vi "BG_move.vi"(4 "Reset_x":i32, 6 "Return_x":i32, 7 "Mov_Spd":i32, 8 "error in":errorcluster, 11 "BG_ref":refnum<vi>[](array[refnum])) -> (0 "error out":errorcluster)   [LabVIEW 8.6]
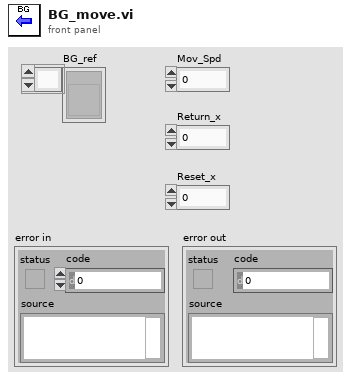
[diagram p1: front panel]
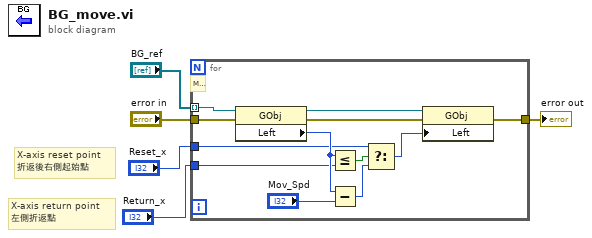
[diagram p0: block diagram]
diagram:
  # "Missing object. The object \"Parallel Instances\" does not exist in the previous version."
  # "X-axis reset point\n折返後右側起始點"
  # "X-axis return point\n左側折返點"
  n1 = for {
    tunnel: "error in" -> [w17]
    tunnel: [w10] -> w4
    tunnel: "BG_ref" -> [w9] mode=indexing
    tunnel: "Return_x" -> [w8]
    tunnel: "Reset_x" -> [w7]
    n2 = property on="Property Node" class="GObj"(reference=w9, error in=w17) -> (reference out=w11:refnum<vi>, error out=w6:errorcluster, "Left"=w15:i32)
    n3 = Less Or Equal?(x=w15, y=w8) -> (x <= y?=w13:bool)
    n4 = Subtract(x=w15, y="Mov_Spd") -> (x-y=w12:i32)
    n5 = Select(t=w7, s=w13, f=w12) -> (s? t:f=w16:i32)
    n6 = property on="Property Node" class="GObj"(reference=w11, error in=w6, "Left"=w16) -> (error out=w10:errorcluster)  [unwired: 1 out]
  }
  "error out" <- w4
